vi "Unit Converter v1.00.vi"(0 "Wavelength Unit":i32(ring)=1 items=["Point #", "nm", "eV", "meV", "cm-1"], 1 "x to W (F) or W to x (T)":bool, 2 "Update?":bool=TRUE, 5 "Grating Density":u8(ring)=2 items=["150 g/mm", "300 g/mm", "600 g/mm", "1200 g/mm", "1800 g/mm"], 7 "Velocity (Steps/s)":i32=42372, 9 "Stepper Position Input":i32 min=-8388607 max=8388607, 12 "Wavelength Input":dbl format="%.2f") -> (3 "Precision":i32, 4 "Wavelength Output":dbl format="%.2f", 6 "Current Couter Position":dbl format="%.2f", 8 "nm Output":dbl format="%.2f", 10 "Slew Rate":dbl format="%.2f", 13 "X-Axis Unit String":string, 14 "UnitFormatString":string="nm", 15 "Stepper Position Output":i32 min=-8388607 max=8388607)   [LabVIEW 2025]
doc: "(1) Convert stepper position to its corresponding wavelength (in the given unit and grating setting)\n(2) Vice versa.\nAuthor: Scott Hannahs <sth@magnet.fsu.edu>\n\nThis software is licensed for use under the “MIT License\"\nCopyright (c) 2025 Scott Hannahs, sth@sth@magnet.sthnet.net\n\nPermission is hereby granted, free of charge, to any person obtaining a copy of this software and associated documentation files (the \"Software\"), to deal in the Software without restriction, including without limitation the rights to use, copy, modify, merge, publish, distribute, sublicense, and/or sell copies of the Software, and to permit persons to whom the Software is furnished to do so, subject to the following conditions: The above copyright notice and this permission notice shall be included in all copies or substantial portions of the Software.\n\nTHE SOFTWARE IS PROVIDED \"AS IS\", WITHOUT WARRANTY OF ANY KIND, EXPRESS OR IMPLIED, INCLUDING BUT NOT LIMITED TO THE WARRANTIES OF MERCHANTABILITY, FITNESS FOR A PARTICULAR PURPOSE AND NONINFRINGEMENT. IN NO EVENT SHALL THE AUTHORS OR COPYRIGHT HOLDERS BE LIABLE FOR ANY CLAIM, DAMAGES OR OTHER LIABILITY, WHETHER IN AN ACTION OF CONTRACT, TORT OR OTHERWISE, ARISING FROM, OUT OF OR IN CONNECTION WITH THE SOFTWARE OR THE USE OR OTHER DEALINGS IN THE SOFTWARE."
uses:
  Globals and TypeDefs/Global Varibal Control.vi
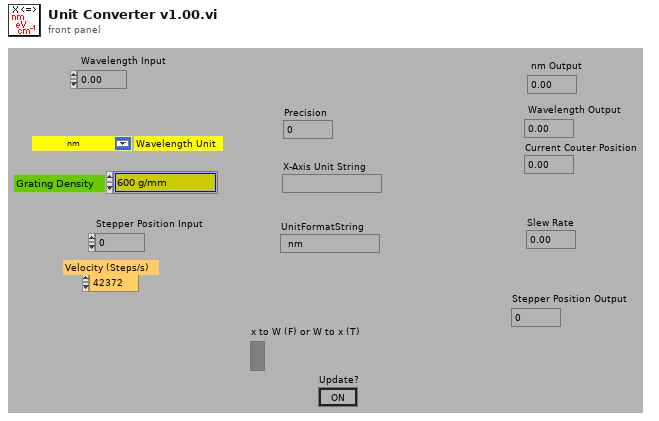
[diagram p1: front panel]
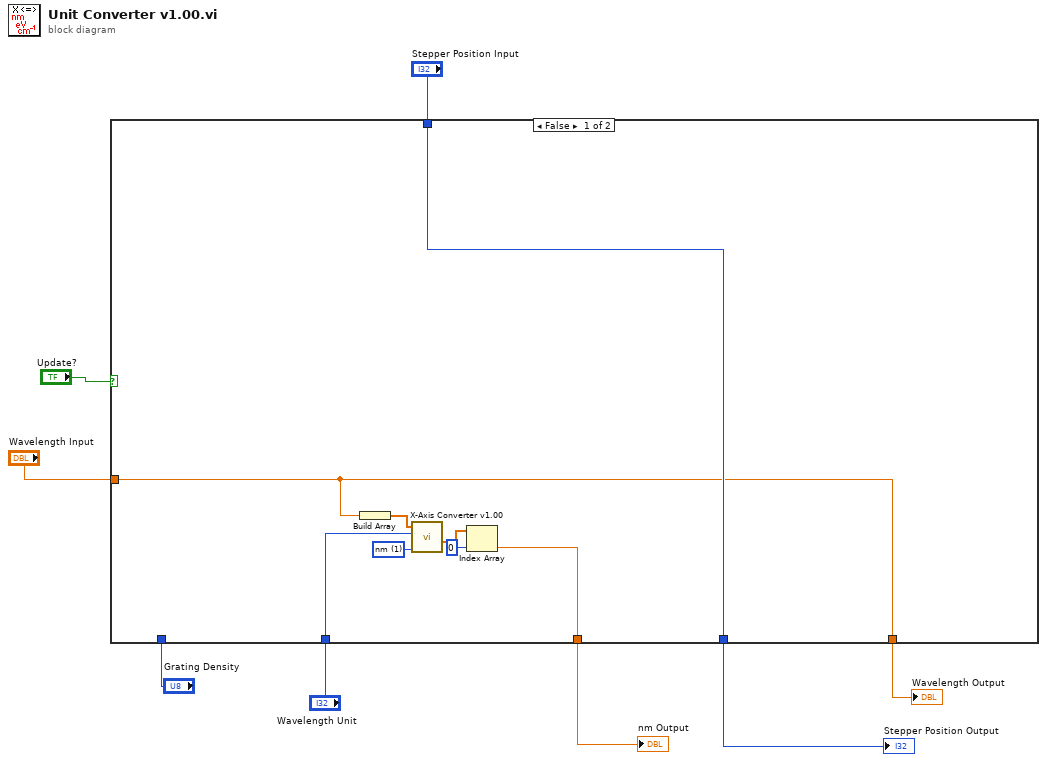
[diagram p0: block diagram]
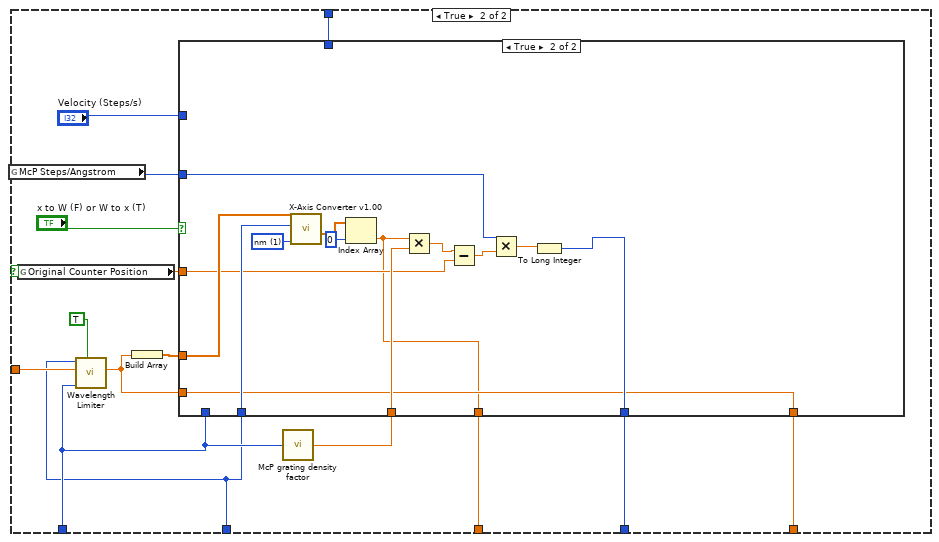
[diagram p2: hidden frame]
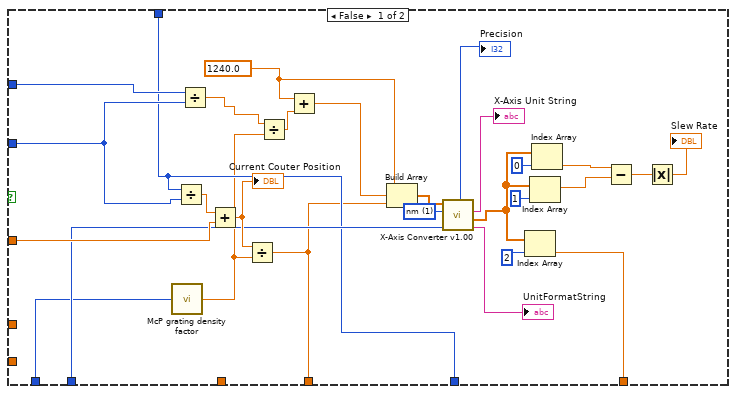
[diagram p3: hidden frame]
diagram:
  n1 = case shown="False" "Update?" {
    tunnel: [w16 w24] -> w8
    tunnel: "Stepper Position Input" -> [w16 w22]
    tunnel: "Wavelength Input" -> [w10 w21]
    tunnel: [w10 w23] -> w4
    tunnel: [w11 w19] -> w3
    tunnel: "Grating Density" -> [_ w18]
    tunnel: "Wavelength Unit" -> [w12 w17]
    frame False {
      w15 = 1 items=["Point #", "nm", "eV", "meV", "cm-1"] ("X-Axis Unit")
      n2 = Build Array(w10) -> (w9:dbl[])
      n3 = call "X-Axis Converter v1.00.vi"("X-Axis Unit"=w15, "Old X-Axis Unit"=w12, "X-Axis input"=w9) -> ("X-Axis Output"=w14:dbl[])  [unwired: 2 in, 3 out]
      n4 = Index Array(array=w14, index=0 ("Index")) -> (element=w11:dbl)
    }
    frame True {
      n5 = global read "Global Varibal Control.vi" "McP Steps/Angstrom"() -> (w30:i32)
      n6 = global read "Global Varibal Control.vi" "Original Counter Position"() -> (w31:dbl)
      n7 = call "Wavelength Limiter.vi"("Range Limiter(F) or WL limiter"=TRUE, "Current Grating Density"=w18, "Central WL Input"=w21, "X-Axis"=w17) -> ("Central WL output"=w20:dbl)  [unwired: 1 in, 3 out]
      n8 = Build Array(w20) -> (w27:dbl[])
      n9 = call "McP grating density factor.vi"("Grating Density"=w18) -> ("GratingFactor"=w25:dbl)
      n10 = case shown="True" "x to W (F) or W to x (T)" {
        tunnel: w31 -> [w42 w66]
        tunnel: w30 -> [w41 w65]
        tunnel: "Velocity (Steps/s)" -> [w40 _]
        tunnel: w18 -> [w38 _]
        tunnel: w17 -> [w39 w73]
        tunnel: w27 -> [_ w71]
        tunnel: w25 -> [_ w68]
        tunnel: [w36 w62] -> w24
        tunnel: [w37 w61] -> w23
        tunnel: w22 -> [w36 _]
        tunnel: w20 -> [_ w61]
        tunnel: [w32 w60] -> w19
        frame False {
          w54 = 1240.0 ("x")
          w56 = 1 items=["Point #", "nm", "eV", "meV", "cm-1"] ("Old X-Axis Unit")
          n11 = call "McP grating density factor.vi"("Grating Density"=w38) -> ("GratingFactor"=w34:dbl)
          n12 = Divide(x=w36, y=w41) -> (x/y=w59:dbl)
          n13 = Divide(x=w40, y=w41) -> (x/y=w33:dbl)
          n14 = Add(x=w59, y=w42) -> (x+y=w58:dbl)
          "Current Couter Position" <- w58
          n15 = Divide(x=w58, y=w34) -> (x/y=w32:dbl)
          n16 = Divide(x=w33, y=w34) -> (x/y=w35:dbl)
          n17 = Add(x=w54, y=w35) -> (x+y=w53:dbl)
          n18 = Build Array(w54, w53, w32) -> (w57:dbl[])
          n19 = call "X-Axis Converter v1.00.vi"("X-Axis Unit"=w39, "Old X-Axis Unit"=w56, "X-Axis input"=w57) -> ("UnitFormatString"=→"UnitFormatString":string, "X-Axis Output"=w52:dbl[], "X-Axis Unit String"=→"X-Axis Unit String":string, "Precision"=→"Precision":i32)  [unwired: 2 in]
          n20 = Index Array(array=w52, index=2 ("Index")) -> (element=w37:dbl)
          n21 = Index Array(array=w52, index=1 ("Index")) -> (element=w45:dbl)
          n22 = Index Array(array=w52, index=0 ("Index")) -> (element=w46:dbl)
          n23 = Subtract(x=w46, y=w45) -> (x-y=w48:dbl)
          n24 = Absolute Value(x=w48) -> (abs(x)=→"Slew Rate":dbl)
        }
        frame True {
          w72 = 1 items=["Point #", "nm", "eV", "meV", "cm-1"] ("X-Axis Unit")
          n25 = call "X-Axis Converter v1.00.vi"("X-Axis Unit"=w72, "Old X-Axis Unit"=w73, "X-Axis input"=w71) -> ("X-Axis Output"=w70:dbl[])  [unwired: 2 in, 3 out]
          n26 = Index Array(array=w70, index=0 ("Index")) -> (element=w60:dbl)
          n27 = Multiply(x=w60, y=w68) -> (x*y=w67:dbl)
          n28 = Subtract(x=w67, y=w66) -> (x-y=w64:dbl)
          n29 = Multiply(x=w65, y=w64) -> (x*y=w63:dbl)
          n30 = To Long Integer(number=w63) -> (32bit integer=w62:i32)
        }
      }
    }
  }
  "Stepper Position Output" <- w8
  "Wavelength Output" <- w4
  "nm Output" <- w3
